vi "Matches.vi"(8 "error in (no error)":errorcluster, 10 "Actual":variant, 11 "ErrorCode in":refnum<class "ErrorCode.lvclass">) -> (0 "error out":errorcluster, 2 "Result":bool, 3 "ErrorCode out":refnum<class "ErrorCode.lvclass">)   [LabVIEW 2017, in "Transparent Assertions.lvlib" / "ErrorCode.lvclass"]
doc: "Evaluates the constraint for <B>Actual</B>. Returns true if the constraint is met."
uses:
  ErrorCode.lvclass
  ErrorCode.lvclass/ErrorCode.ctl
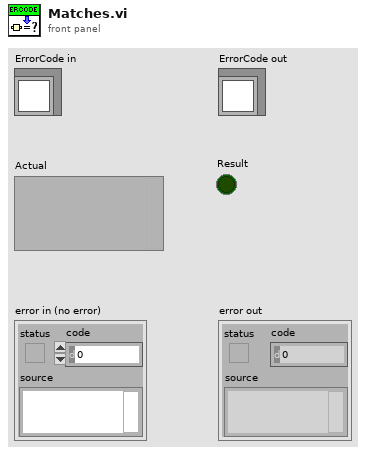
[diagram p1: front panel]
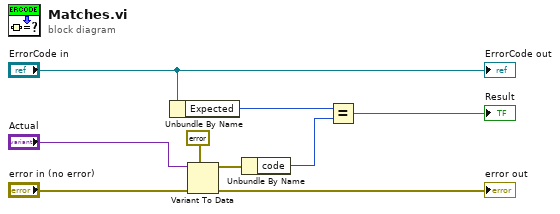
[diagram p0: block diagram]
diagram:
  n1 = Unbundle By Name("ErrorCode in") -> ("Expected"=w2:i32)
  n2 = Variant To Data(error in="error in (no error)", type=errorcluster {"status"=FALSE, "code"=0, "source"=""} ("error constant"), Variant="Actual") -> (data=w5:errorcluster, error out=→"error out":errorcluster)
  n3 = Unbundle By Name(w5) -> ("code"=w3:i32)
  n4 = Equal?(x=w2, y=w3) -> (x = y?=→"Result":bool)
  "ErrorCode out" <- "ErrorCode in"
